vi "GSI-HVSwitch2.set voltage steps.vi"(0 "i ref in":refnum<vi>, 2 "voltageSteps [V]":dbl[](array[numeric]), 3 "ms timeout (10000)":i32=10000, 5 "error in (no error)":errorcluster) -> (14 "i ref out":refnum<vi>, 17 "timed out":bool, 19 "error out":errorcluster)   [LabVIEW 2014, in "GSI-HVSwitch2.lvlib"]
doc: "Loads an array of voltage steps to the device. Don't use the method while the device is triggered."
uses:
  GSI-HVSwitch2.lvlib
  CSCore/CSApplicationBaseClasses/PSChannelBase/PSChannelBase.directionType.ctl
  CSCore/CSApplicationBaseClasses/PSChannelBase/PSChannelBase.serviceType.ctl
  CSlibraries/UtilityLib/UtilityLib.valueStatus.ctl
  CSCore/CSApplicationBaseClasses/DeviceBase/DeviceBase.deviceState.ctl
  CSCore/CSSystem/CoreDefs/CoreDefs.error_type.ctl
  CSCore/CSSystem/CoreDefs/CoreDefs.error_severity.ctl
  CSCore/CSSystem/CoreLib/CoreLib.lvlib
  CSCore/CSApplicationBaseClasses/PSChannelBase/PSChannelBase.lvlib
  CSlibraries/UtilityLib/UtilityLib.lvlib
  CSCore/CSApplicationBaseClasses/DeviceBase/DeviceBase.lvlib
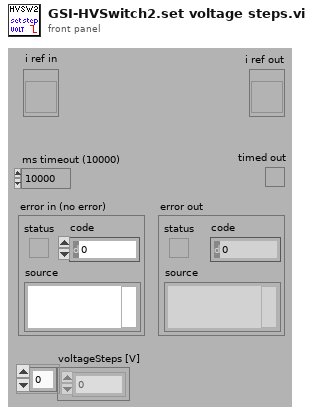
[diagram p1: front panel]
types:
  T1 = typedef "UtilityLib.lvlib/UtilityLib.valueStatus.ctl" = enum16{"no info available", "stand by/off", "on", "warning", "alarm/malfunction", "not implemented", "user action required", "important information", "system default", "control default", "indicator default", "button default"}
  T2 = typedef "PSChannelBase.lvlib/PSChannelBase.serviceType.ctl" = enum16{"onOff", "voltage", "current", "tripCurrent", "rampUpSpeed", "rampDownSpeed", "status"}
  T3 = typedef "PSChannelBase.lvlib/PSChannelBase.directionType.ctl" = enum16{"unknown", "update actual value", "update nominal value", "update both"}
  T4 = typedef "CoreDefs.error_severity.ctl" = enum16{"undefined", "information", "warning", "error", "fatal"}
  T5 = typedef "CoreDefs.error_type.ctl" = enum16{"no error", "can't load process", "can't unload process", "process does not exist", "can't install process", "can't remove process", "unknown function", "time out", "can't execute function", "duplicate queue name", "super not found", "caller queue invalid", "can't ping process", "unknown error", "VISA Error", "VISA timeout", "GPIB timeout", "GPIB error", "communication error", "data type mismatch", "can't read data from OPC server", "can't write data to OPC server", "OET error", "function not implemented", "process already exists", "invalid Shared Variable name", "error writing Shared Variable", "error reading Shared Variable", "invalid client name", "corrupt database", "unknown class", "call not authorized", "parameter out of range", "OET timeout: can't get data to modify", "invalid queue name", "requested operation incompatible with current state", "event undefined", "event disabled", "state undefined", "caller is not a friend", "EventBuilder: bad eventID", "EventBuilder: no DAQ devices", "a thread must not stop itself", "UNUSED ELEMENT4", "DiscArchiver: eventData incomplete", "DiscArchiver: eventData does not belong to run", "DiscArchiver: can't open file", "DiscArchiver: can't write to file", "DiscArchiver: available disc space low", "can't acquire semaphore", "error reading data from database", "notifier object is not existing", "can't register process", "can't unregister process", "illegal event type", "object disabled", "object already exists", "can't change state", "Instrument not found", "no connection to remote node", "invalid reference", "N/A", "UNUSED ELEMENT 1", "element not found", "illegal TCP/IP connection detected", "object does not exist", "invalid access ID", "unknown CS system", "invalid privilige", "unsupported data type", "unsupported server type", "IO server already exists", "Shared Variable already exists"}
  T6 = typedef "DeviceBase.lvlib/DeviceBase.deviceState.ctl" = i16
  T7 = typedef "GSI-HVSwitch2.lvlib/GSI-HVSwitch2.i attribute.ctl" = cluster{"SDEX VISA Cluster":T8, "SetVoltage SW0":dbl, "SetVoltage SW1":dbl, "ActTempAmp":dbl, "ActTempPS1":dbl, "ActTempPS2":dbl, "mode":T11, "interfaceInitialized":bool, "serviceIDs":cluster{"nomVoltage0ID":i32, "nomVoltage1ID":i32, "actTempAmpID":i32, "actTempPS1ID":i32, "actTempPS2ID":i32, "modeID":i32}, "usedChannels":i32}
  T8 = typedef "SDEXDriver.lvlib/SDEX.VISA Control.ctl" = cluster{"VISA resource name":refnum<visa-resource-name>, "HEX address":u16, "VISA Timeout Value (1000 ms)":u32, "Lock Timeout (1000 ms)":u32, "semaphore":T9, "Baud rate":u32, "revision":T10, "deviceInfo":string}
  T9 = typedef "Semaphore RefNum" = refnum<k1>
  T10 = typedef "SDEXDriver.lvlib/SDEX.revisionType.ctl" = enum16{"unknown", "hvamp3", "hvswi1", "htrp0", "WDG0"}
  T11 = typedef "GSI-HVSwitch2.lvlib/GSI-HVSwitch2.mode.ctl" = enum16{"unknown", "switch", "stepper"}
  T12 = typedef "PSChannelBase.lvlib/PSChannelBase.i attribute.ctl" = cluster{"defaultChannelIndex":i32, "nofChannels":i32, "defaultChannelIndexID":i32, "nofChannelsID":i32, "actValues":T13, "nomValues":T13, "logicalName":string[], "physicalName":string[], "logicalNameID":i32, "physicalNameID":i32}
  T13 = typedef "PSChannelBase.lvlib/PSChannelBase.parameters.ctl" = cluster{"onOff":bool[], "voltage":dbl[], "current":dbl[], "tripCurrent":dbl[], "rampUpSpeed":dbl[], "rampDownSpeed":dbl[], "status":i32[], "serviceIDs":cluster{"onOfflID":i32, "voltageID":i32, "currentID":i32, "tripCurrentID":i32, "rampUpSpeedID":i32, "rampDownSpeedID":i32, "statusID":i32}}
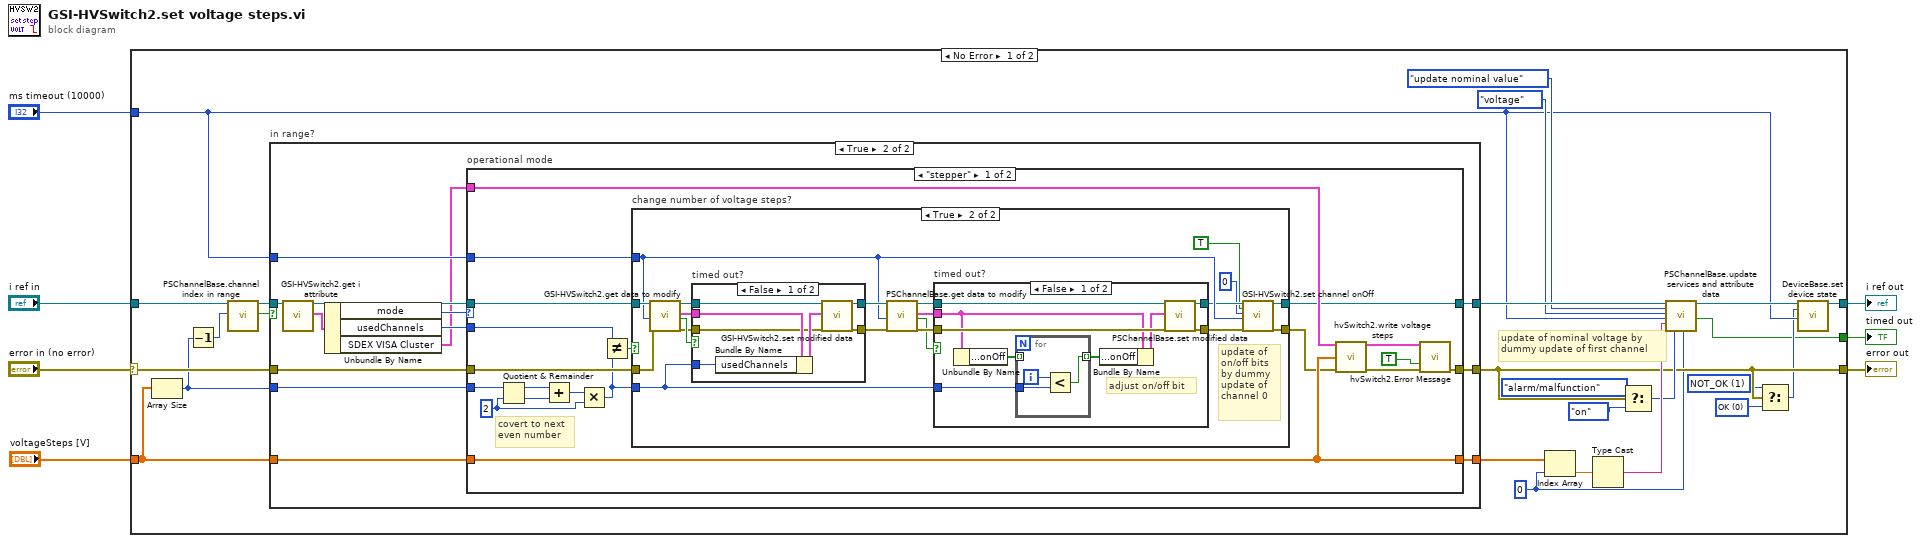
[diagram p0: block diagram]
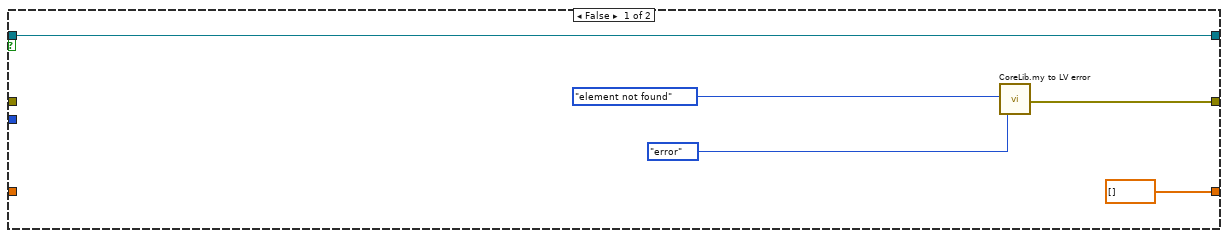
[diagram p2: hidden frame]
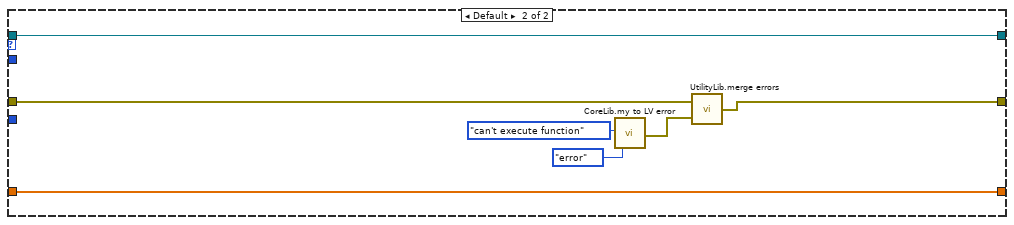
[diagram p6: hidden frame]
diagram:
  n1 = case shown="No Error" "error in (no error)" {
    selector: "error in (no error)" -> [w32 w122]
    tunnel: "i ref in" -> [w17 w123]
    tunnel: "ms timeout (10000)" -> [w22 _]
    tunnel: [w9 _] -> w5
    tunnel: [w23 w123] -> w4
    tunnel: [w21 w122] -> w3
    tunnel: "voltageSteps [V]" -> [w13 _]
    frame No Error {
      w19 = T6 1 items=["ERROR"=-1, "OK"=0, "NOT_OK"=1] ("deviceState")
      w20 = T6 0 items=["ERROR"=-1, "OK"=0, "NOT_OK"=1] ("deviceState")
      w10 = 0 ("index")
      # "update of nominal voltage by\ndummy update of first channel"
      n2 = Array Size(array=w13) -> (size(s)=w8:i32)
      n3 = Decrement(x=w8) -> (x-1=w11:i32)
      n4 = call "PSChannelBase.channel index in range.vi"("i ref in"=w17, "channelIndex"=w11) -> ("i ref out"=w16:refnum<vi>, "in range"=w15:bool)  [unwired: 15 in, 1 out]
      n5 = case "in range?" shown="True" w15 {
        tunnel: w16 -> [w35 w46]
        tunnel: w22 -> [_ w50]
        tunnel: [w35 w47] -> w31
        tunnel: [w34 w49] -> w21
        tunnel: w32 -> [_ w48]
        tunnel: w13 -> [_ w39]
        tunnel: [dbl[] [] ("voltageSteps [V]") w42] -> w14
        tunnel: w8 -> [_ w38]
        frame False {
          n6 = call "CoreLib.my to LV error.vi"("ErrorTypes"=CoreDefs.error_type."element not found", "severityLevel"=CoreDefs.error_severity."error") -> ("myErrorCluster"=w34:errorcluster)  [unwired: 16 in, 1 out]
        }
        frame True {
          n7 = call "GSI-HVSwitch2.get i attribute.vi"("i ref in"=w46) -> ("i ref out"=w43:refnum<vi>, "i attribute"=w45:T7)  [unwired: 16 in, 1 out]
          n8 = Unbundle By Name(w45) -> ("mode"=w44:T11, "usedChannels"=w41:i32, "SDEX VISA Cluster"=w40:T8)
          n9 = case "operational mode" shown="\"stepper\"" w44 {
            tunnel: w50 -> [w66 _]
            tunnel: [w64 w117] -> w49
            tunnel: w48 -> [w68 w119]
            tunnel: [w57 w116] -> w47
            tunnel: w38 -> [w56 _]
            tunnel: w39 -> [w59 w115]
            tunnel: w43 -> [w69 w116]
            tunnel: [w59 w115] -> w42
            tunnel: w41 -> [w65 _]
            tunnel: w40 -> [w61 _]
            frame "stepper" {
              w52 = 2 ("y")
              # "covert to next \neven number"
              n10 = Quotient & Remainder(x=w56, y=w52) -> (x-y*floor(x/y)=w55:i32, floor(x/y)=w54:i32)
              n11 = Add(x=w55, y=w54) -> (x+y=w53:i32)
              n12 = Multiply(x=w53, y=w52) -> (x*y=w51:i32)
              n13 = Not Equal?(x=w65, y=w51) -> (x != y?=w67:bool)
              n14 = case "change number of voltage steps?" shown="True" w67 {
                tunnel: w69 -> [w70 w91]
                tunnel: w68 -> [w71 w90]
                tunnel: [w70 w73] -> w57
                tunnel: [w71 w72] -> w58
                tunnel: w51 -> [_ w79]
                tunnel: w66 -> [_ w78]
                frame False {
                }
                frame True {
                  # "update of\non/off bits\nby dummy\nupdate of\nchannel 0"
                  n15 = call "GSI-HVSwitch2.get data to modify.vi"("i ref in"=w91, "ms timeout (10000)"=w78, "error in (no error)"=w90) -> ("i ref out"=w88:refnum<vi>, "i attribute"=w86:T7, "timed out"=w89:bool, "error out"=w87:errorcluster)  [unwired: 13 in]
                  n16 = case "timed out?" shown="False" w89 {
                    tunnel: w88 -> [w107 w114]
                    tunnel: [w112 w114] -> w84
                    tunnel: w87 -> [w108 w113]
                    tunnel: [w111 w113] -> w85
                    tunnel: w86 -> [w109 _]
                    tunnel: w79 -> [w106 _]
                    frame False {
                      n17 = Bundle By Name(cluster=w109, "usedChannels"=w106) -> (w110:T7)
                      n18 = call "GSI-HVSwitch2.set modified data.vi"("i ref in"=w107, "i attribute"=w110, "error in (no error)"=w108) -> ("i ref out"=w112:refnum<vi>, "error out"=w111:errorcluster)  [unwired: 15 in]
                    }
                    frame True {
                    }
                  }
                  n19 = call "PSChannelBase.get data to modify.vi"("i ref in"=w84, "ms timeout (10000)"=w78, "error in (no error)"=w85) -> ("i ref out"=w83:refnum<vi>, "i attribute"=w80:T12, "timed out"=w81:bool, "error out"=w82:errorcluster)  [unwired: 13 in]
                  n20 = case "timed out?" shown="False" w81 {
                    tunnel: w83 -> [w100 w105]
                    tunnel: [w99 w105] -> w77
                    tunnel: [w98 w104] -> w76
                    tunnel: w82 -> [w97 w104]
                    tunnel: w80 -> [w96 _]
                    tunnel: w79 -> [w94 _]
                    frame False {
                      # "adjust on/off bit"
                      n21 = Unbundle By Name(w96) -> ("nomValues.onOff"=w95:bool[])
                      n22 = for {
                        tunnel: w95 -> [_] mode=indexing
                        tunnel: w94 -> [w102]
                        tunnel: [w101] -> w93 mode=indexing
                        i -> [w103]
                        n23 = Less?(x=w103, y=w102) -> (x < y?=w101:bool)
                      }
                      n24 = Bundle By Name(cluster=w96, "nomValues.onOff"=w93) -> (w92:T12)
                      n25 = call "PSChannelBase.set modified data.vi"("i ref in"=w100, "i attribute"=w92, "error in (no error)"=w97) -> ("i ref out"=w99:refnum<vi>, "error out"=w98:errorcluster)  [unwired: 15 in]
                    }
                    frame True {
                    }
                  }
                  n26 = call "GSI-HVSwitch2.set channel onOff.vi"("i ref in"=w77, "on (FALSE)"=TRUE, "channel"=0, "ms timeout (10000)"=w78, "error in (no error)"=w76) -> ("i ref out"=w73:refnum<vi>, "error out"=w72:errorcluster)  [unwired: 12 in, 1 out]
                }
              }
              n27 = call "hvSwitch2.write voltage steps.vi"("SDEX VISA Cluster"=w61, "voltageSteps"=w59, "error in (no error)"=w58) -> ("dup SDEX VISA Cluster"=w60:T8, "error out"=w62:errorcluster)  [unwired: 11 in]
              n28 = call "hvSwitch2.Error Message.vi"("SDEX VISA Cluster"=w60, "append msg 2 src"=TRUE, "error in (no error)"=w62) -> ("error out"=w64:errorcluster)  [unwired: 8 in, 4 out]
            }
            frame Default {
              n29 = call "CoreLib.my to LV error.vi"("ErrorTypes"=CoreDefs.error_type."can't execute function", "severityLevel"=CoreDefs.error_severity."error") -> ("myErrorCluster"=w118:errorcluster)  [unwired: 16 in, 1 out]
              n30 = call "UtilityLib.merge errors.vi"("error2 (no error)"=w118, "error1 (no error)"=w119) -> ("error out"=w117:errorcluster)
            }
          }
        }
      }
      n31 = Index Array(array=w14, index=w10) -> (element=w12:dbl)
      n32 = Type Cast(x=w12) -> (*(type *) &x=w28:string)  [unwired: 1 in]
      n33 = Select(t=UtilityLib.valueStatus."alarm/malfunction" ("quality"), s=w21, f=UtilityLib.valueStatus."on") -> (s? t:f=w25:T1)
      n34 = call "PSChannelBase.update services and attribute data.vi"("i ref in"=w31, "direction"=PSChannelBase.directionType."update nominal value", "service"=PSChannelBase.serviceType."voltage", "ms timeout (10000)"=w22, "value"=w28, "quality"=w25, "channelNumber"=w10) -> ("i ref out"=w24:refnum<vi>, "timed out"=w9:bool)  [unwired: 10 in, 1 out]
      n35 = Select(t=w19, s=w21, f=w20) -> (s? t:f=w18:T6)
      n36 = call "DeviceBase.set device state.vi"("i ref in"=w24, "deviceState"=w18, "ms timeout (10000)"=w22) -> ("i ref out"=w23:refnum<vi>)  [unwired: 14 in, 2 out]
    }
    frame Error {
    }
  }
  "error out" <- w3
  "i ref out" <- w4
  "timed out" <- w5
